vi "Lineas.vi"   [LabVIEW 2017]
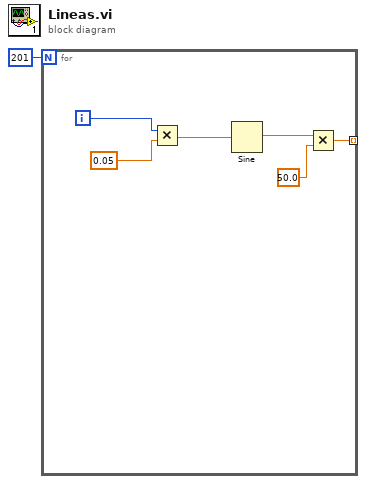
[diagram p0: block diagram]
diagram:
  n1 = for {
    N: 201 -> [_]
    tunnel: [w2] -> _ mode=indexing
    i -> [w6]
    n2 = Multiply(x=w6, y=0.05) -> (x*y=w5:dbl)
    n3 = Sine(x=w5) -> (sin(x)=w4:dbl)
    n4 = Multiply(x=w4, y=50.0) -> (x*y=w2:dbl)
  }
